vi "GetCurrent.vi"(4 "error in":errorcluster, 5 "connection ID":refnum<k5>) -> (0 "Current":string, 1 "error out":errorcluster, 2 "connection ID out":refnum<k5>, 3 "Answer":bool)   [LabVIEW 2013]
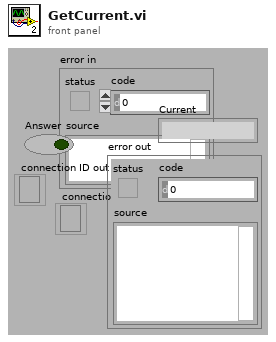
[diagram p1: front panel]
types:
  T1 = enum16{"Standard", "Buffered", "CRLF", "Immediate"}
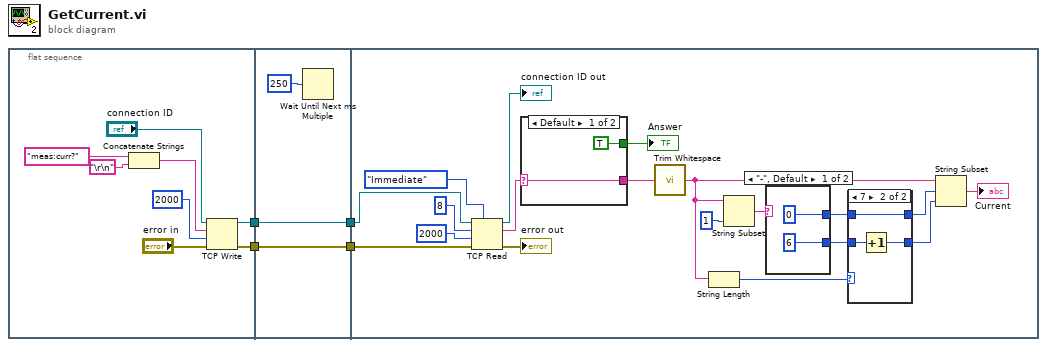
[diagram p0: block diagram]
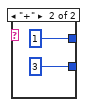
[diagram p3: hidden frame]
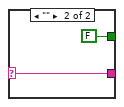
[diagram p4: hidden frame]
diagram:
  n1 = flat-sequence {
    tunnel: [w9] -> w3
    tunnel: [w8] -> w1
    tunnel: [w14] -> w4
    tunnel: w3 -> [w14]
    tunnel: [w13] -> w2
    tunnel: w1 -> [w13]
    tunnel: w4 -> [w27]
    tunnel: w2 -> [w26]
    frame #0 {
      n2 = Concatenate Strings("meas:curr?" ("data in"), "\r\n") -> (w6:string)
      n3 = TCP Write(connection ID="connection ID", data in=w6, error in (no error)="error in", 9:2000 ("timeout ms (25000)")) -> (connection ID out=w9:refnum<k5>, error out=w8:errorcluster)  [unwired: 1 out]
    }
    frame #1 {
      n4 = Wait Until Next ms Multiple(millisecond multiple=u32 250) -> ()  [unwired: 1 out]
    }
    frame #2 {
      n5 = TCP Read(connection ID=w27, bytes to read=8, error in (no error)=w26, 7:T1."Immediate" ("mode (standard)"), 9:2000 ("timeout ms (25000)")) -> (connection ID out=→"connection ID out":refnum<k5>, data out=w32:string, error out=→"error out":errorcluster)
      n6 = case shown="Default" w32 {
        selector: w32 -> [w45 w47]
        tunnel: [w45 w47] -> w17
        tunnel: [TRUE FALSE] -> w31
        frame Default {
        }
        frame "" {
        }
      }
      "Answer" <- w31
      n7 = call <vilib>:"Trim Whitespace.vi"("string"=w17) -> ("trimmed string"=w20:string)  [unwired: 1 in]
      n8 = String Length(string=w20) -> (length=w21:i32)
      n9 = String Subset(string=w20, length (rest)=1 ("length (rest)")) -> (substring=w18:string)  [unwired: 1 in]
      n10 = case shown="\"-\", Default" w18 {
        tunnel: [0 ("length (rest)") 1 ("length (rest)")] -> w24
        tunnel: [6 ("length (rest)") 3 ("length (rest)")] -> w22
        frame "-", Default {
        }
        frame "+" {
        }
      }
      n11 = case shown="7" w21 {
        tunnel: w22 -> [w36 w39]
        tunnel: [w36 w38] -> w23
        tunnel: w24 -> [w35 w37]
        tunnel: [w35 w37] -> w25
        frame 6, Default {
        }
        frame 7 {
          n12 = Increment(x=w39) -> (x+1=w38:i32)
        }
      }
      n13 = String Subset(string=w20, offset (0)=w25, length (rest)=w23) -> (substring=→"Current":string)
    }
  }
